vi "test_md5.vi"() -> (3 "All Passed?":bool)   [LabVIEW 2021]
uses:
  src/hashlib.lvlib
panel:
  in  "Data in":T1(array[cluster])=[{"String"="The dog jumped over the river", "MD5 (Hex String)"="a6aa051024f546143498bd5121b13a7d", "MD5 (16-bytes)"="¦ª\u0005\u0010$õF\u00144˜½Q!±:}"}, {"String"="\u0000", "MD5 (Hex String)"="93b885adfe0da089cdf634904fd59f71", "MD5 (16-bytes)"="¸­þ\r Íö4OÕq"}, {"String"="\u0001\u0002\u0003\ff", "MD5 (Hex String)"="00e76eeb40eca625c8499aeabcd3c0d0", "MD5 (16-bytes)"="\u0000çnë@ì¦%ÈIšê¼ÓÀÐ"}, {"String"="", "MD5 (Hex String)"="d41d8cd98f00b204e9800998ecf8427e", "MD5 (16-bytes)"="Ô\u001dÙ\u0000²\u0004é\tìøB~"}]
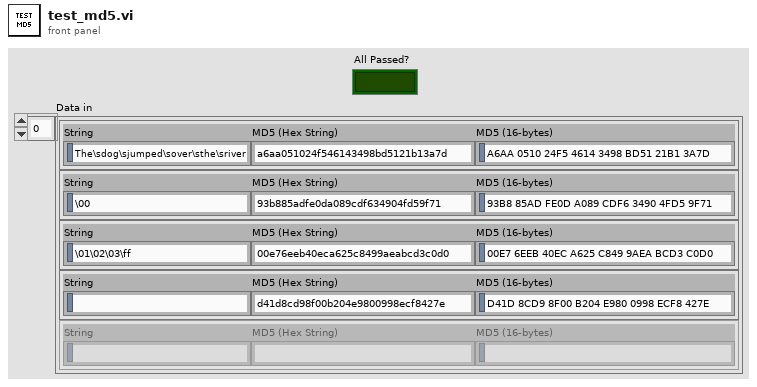
[diagram p1: front panel]
types:
  T1 = cluster{"String":string, "MD5 (Hex String)":string, "MD5 (16-bytes)":string}[]
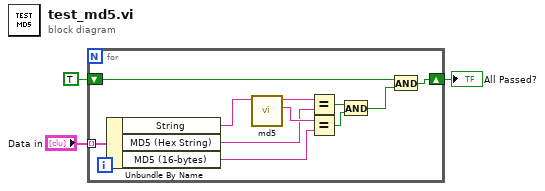
[diagram p0: block diagram]
diagram:
  n1 = for {
    shift-right: [w13] -> w2
    shift-left: TRUE -> [w14]
    tunnel: "Data in" -> [w12] mode=indexing
    n2 = Unbundle By Name(w12) -> ("String"=w11:string, "MD5 (Hex String)"=w5:string, "MD5 (16-bytes)"=w4:string)
    n3 = call "md5.vi"("Data in"=w11) -> ("MD5 (16-bytes)"=w9:string, "MD5 (Hex String)"=w10:string)  [unwired: 9 in]
    n4 = Equal?(x=w10, y=w5) -> (x = y?=w8:bool)
    n5 = Equal?(x=w9, y=w4) -> (x = y?=w7:bool)
    n6 = And(x=w8, y=w7) -> (x .and. y?=w6:bool)
    n7 = And(x=w14, y=w6) -> (x .and. y?=w13:bool)
  }
  "All Passed?" <- w2
